vi "IntakeBegin.vi"(8 "error in (no error)":errorcluster) -> (0 "error out":errorcluster)   [LabVIEW 2023]
uses:
  <vilib>/Rock Robotics/WPI/ThirdParty/REV Robotics/REVLib/Typedef/Spark MAX Idle Mode.ctl
  <vilib>/Rock Robotics/SystemInterfaces/DIO/FPGA_DIOChannel.ctl
  <vilib>/Rock Robotics/WPI/ThirdParty/REV Robotics/REVLib/SubVI/Public/SPARK Open Brushless.vi
  <vilib>/Rock Robotics/WPI/ThirdParty/REV Robotics/REVLib/SubVI/Public/SPARK Configure Basic Idle Mode.vi
  <vilib>/Rock Robotics/WPI/Switch/WPI_SwitchOpenLimit.vi
  <vilib>/Rock Robotics/WPI/ThirdParty/REV Robotics/REVLib/SubVI/Public/SPARK Configure Basic Ramp Rate.vi
  <vilib>/Rock Robotics/WPI/ThirdParty/REV Robotics/REVLib/SubVI/Public/SPARK Configure Power Smart Current Limit.vi
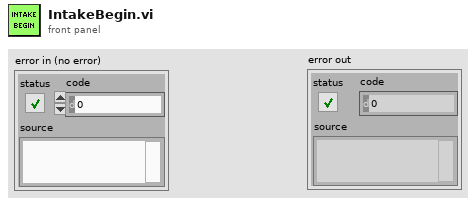
[diagram p1: front panel]
types:
  T1 = typedef "Spark MAX Idle Mode.ctl" = enum16{"Coast", "Brake"}
  T2 = typedef "FPGA_DIOChannel.ctl" = enum8{"DIO 0", "DIO 1", "DIO 2", "DIO 3", "DIO 4", "DIO 5", "DIO 6", "DIO 7", "DIO 8", "DIO 9", "DIO MXP 0", "DIO MXP 1", "DIO MXP 2", "DIO MXP 3", "DIO MXP 4", "DIO MXP 5", "DIO MXP 6", "DIO MXP 7", "DIO MXP 8", "DIO MXP 9", "DIO MXP 10", "DIO MXP 11", "DIO MXP 12", "DIO MXP 13", "DIO MXP 14", "DIO MXP 15", "SPI Port CS1", "SPI Port CS2", "SPI Port CS3", "SPI Port MISO", "SPI Port MOSI", "Invalid"}
  T3 = typedef "WPI_SwitchDevRef.ctl" = cluster{"DevStatus":errorcluster, "DIO Channel":T2, "CntIndex":T4, "Normally Closed":bool}
  T4 = typedef "FPGA_CounterCtrSystemIndex.ctl" = enum8{"Ctr 0", "Ctr 1", "Ctr 2", "Ctr 3", "Ctr 4", "Ctr 5", "Ctr 6", "Ctr 7", "Invalid"}
  T5 = typedef "WPI_MotorControlDeviceRef.ctl" = cluster{"DeviceStatus":errorcluster, "Type":T6, "PWM":cluster{"PWM Channel":T7, "DeadBand":T8}, "CAN":cluster{"Device Number":u8, "SetOutput VI Ref":variant, "GetOutput VI Ref":variant, "Enable VI Ref":variant, "Disable VI Ref":variant, "Data":variant}, "Invert":bool, "DIO PWM":cluster{"PWM \"Enable\" Channel":T7, "DIOChannel":T2, "PWM Rate":dbl}}
  T6 = typedef "WPI_MotorControlType.ctl" = enum16{"PWM", "CAN", "DIO PWM"}
  T7 = typedef "FPGA_DIOPWMChannel.ctl" = enum8{"PWM 0", "PWM 1", "PWM 2", "PWM 3", "PWM 4", "PWM 5", "PWM 6", "PWM 7", "PWM 8", "PWM 9", "PWM MXP 0", "PWM MXP 1", "PWM MXP 2", "PWM MXP 3", "PWM MXP 4", "PWM MXP 5", "PWM MXP 6", "PWM MXP 7", "PWM MXP 8", "PWM MXP 9", "Invalid"}
  T8 = typedef "WPI_PWMDeadband.ctl" = cluster{"Name":string, "maxPositivePwm":i32, "minPositivePwm":i32, "centerPwm":i32, "maxNegativePwm":i32, "minNegativePwm":i32, "angularRange":u16}
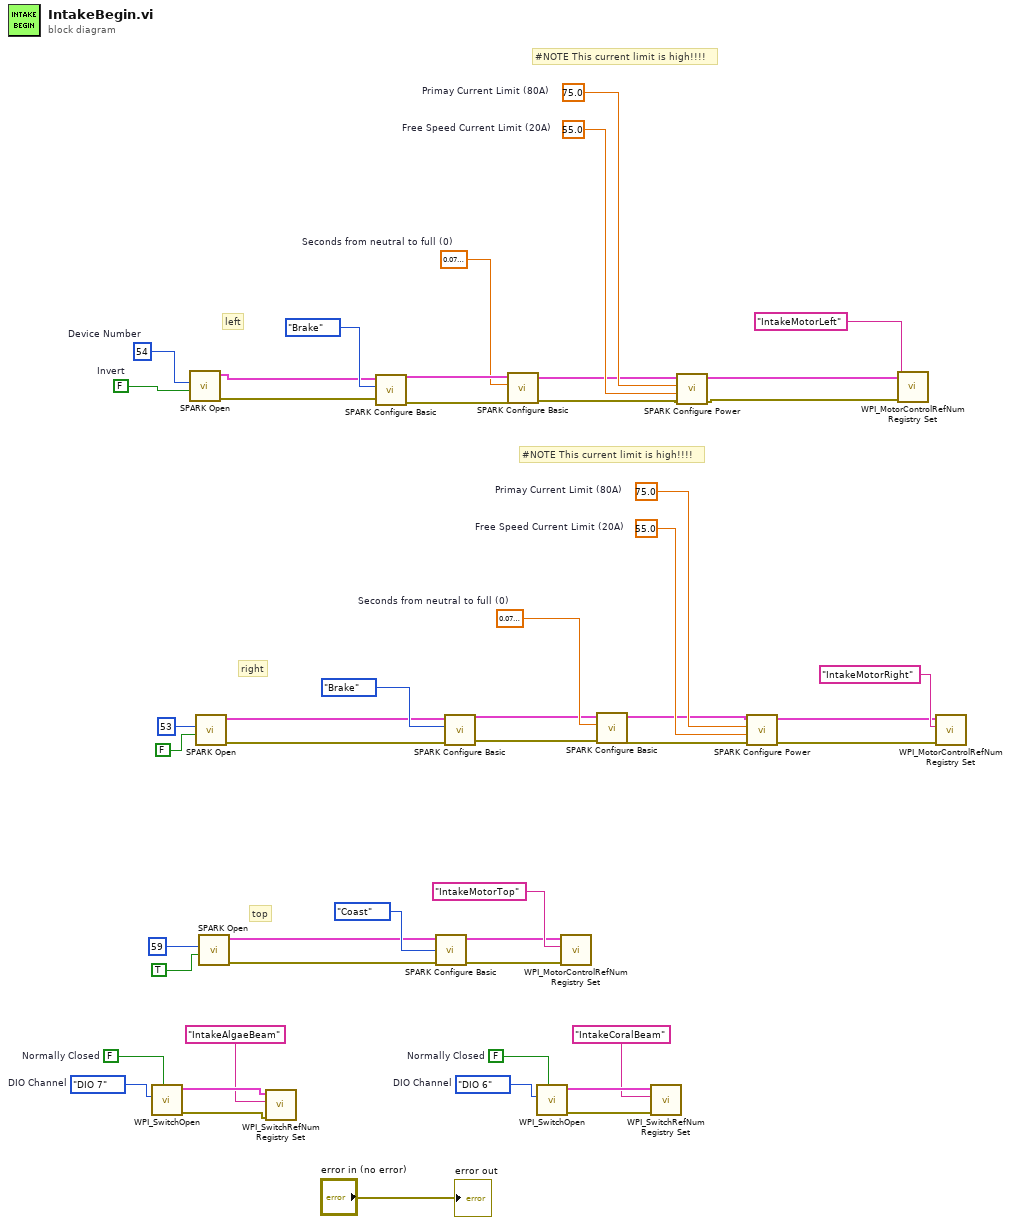
[diagram p0: block diagram]
diagram:
  w13 = sgl 0.08  # Seconds from neutral to full (0)
  w14 = sgl 0.08  # Seconds from neutral to full (0)
  w21 = 55.0  # Free Speed Current Limit (20A)
  w22 = 75.0  # Primay Current Limit (80A)
  w25 = 55.0  # Free Speed Current Limit (20A)
  w26 = 75.0  # Primay Current Limit (80A)
  w30 = FALSE  # Normally Closed
  w31 = FPGA_DIOChannel."DIO 6"  # DIO Channel
  w36 = FALSE  # Normally Closed
  w37 = FPGA_DIOChannel."DIO 7"  # DIO Channel
  w48 = FALSE  # Invert
  w49 = u8 54  # Device Number
  # "top"
  # "#NOTE This current limit is high!!!!"
  # "#NOTE This current limit is high!!!!"
  # "right"
  # "left"
  n1 = call-poly <vilib>:"WPI_SwitchOpen.vi"("Normally Closed"=w36, "DIO Channel"=w37) -> ("error out"=w34:errorcluster, "SwitchDevRef"=w35:T3)  [unwired: 8 in]
  n2 = call-poly <vilib>:"SPARK Open.vi"("Invert"=w48, "Device Number"=w49) -> ("error out"=w40:errorcluster, "MotorControlDeviceRef"=w41:T5)  [unwired: 8 in]
  n3 = call-poly <vilib>:"SPARK Open.vi"("Invert"=FALSE, "Device Number"=u8 53) -> ("error out"=w43:errorcluster, "MotorControlDeviceRef"=w42:T5)  [unwired: 8 in]
  n4 = call-poly <vilib>:"SPARK Open.vi"("Invert"=TRUE, "Device Number"=u8 59) -> ("error out"=w4:errorcluster, "MotorControlDeviceRef"=w5:T5)  [unwired: 8 in]
  n5 = call <vilib>:"WPI_SwitchRefNum Registry Set.vi"("error in (no error)"=w34, "refnum name"="IntakeAlgaeBeam", "SwitchDevRef"=w35) -> ()  [unwired: 7 in, 2 out]
  n6 = call-poly <vilib>:"SPARK Configure Basic.vi"("error in (no error)"=w40, "Idle Mode"=Spark_MAX_Idle_Mode."Brake", "MotorControlDeviceRef in"=w41) -> ("error out"=w17:errorcluster, "MotorControlDeviceRef out"=w18:T5)  [unwired: 7 in]
  n7 = call-poly <vilib>:"SPARK Configure Basic.vi"("error in (no error)"=w4, "Idle Mode"=Spark_MAX_Idle_Mode."Coast", "MotorControlDeviceRef in"=w5) -> ("error out"=w1:errorcluster, "MotorControlDeviceRef out"=w2:T5)  [unwired: 7 in]
  n8 = call-poly <vilib>:"SPARK Configure Basic.vi"("error in (no error)"=w43, "Idle Mode"=Spark_MAX_Idle_Mode."Brake", "MotorControlDeviceRef in"=w42) -> ("error out"=w11:errorcluster, "MotorControlDeviceRef out"=w12:T5)  [unwired: 7 in]
  n9 = call-poly <vilib>:"SPARK Configure Basic.vi"("error in (no error)"=w17, "Seconds from neutral to full (0)"=w14, "MotorControlDeviceRef in"=w18) -> ("error out"=w16:errorcluster, "MotorControlDeviceRef"=w15:T5)  [unwired: 7 in]
  n10 = call-poly <vilib>:"WPI_SwitchOpen.vi"("Normally Closed"=w30, "DIO Channel"=w31) -> ("error out"=w28:errorcluster, "SwitchDevRef"=w29:T3)  [unwired: 8 in]
  n11 = call <vilib>:"WPI_MotorControlRefNum Registry Set.vi"("error in (no error)"=w1, "refnum name"="IntakeMotorTop", "MotorControlDevRef"=w2) -> ()  [unwired: 7 in, 2 out]
  n12 = call-poly <vilib>:"SPARK Configure Basic.vi"("error in (no error)"=w11, "Seconds from neutral to full (0)"=w13, "MotorControlDeviceRef in"=w12) -> ("error out"=w9:errorcluster, "MotorControlDeviceRef"=w10:T5)  [unwired: 7 in]
  n13 = call <vilib>:"WPI_SwitchRefNum Registry Set.vi"("error in (no error)"=w28, "refnum name"="IntakeCoralBeam", "SwitchDevRef"=w29) -> ()  [unwired: 7 in, 2 out]
  n14 = call-poly <vilib>:"SPARK Configure Power.vi"("error in (no error)"=w16, "Free Speed Current Limit (20A)"=w25, "Primay Current Limit (80A)"=w26, "MotorControlDeviceRef in"=w15) -> ("error out"=w23:errorcluster, "MotorControlDeviceRef out"=w24:T5)  [unwired: 6 in]
  n15 = call-poly <vilib>:"SPARK Configure Power.vi"("error in (no error)"=w9, "Free Speed Current Limit (20A)"=w21, "Primay Current Limit (80A)"=w22, "MotorControlDeviceRef in"=w10) -> ("error out"=w19:errorcluster, "MotorControlDeviceRef out"=w20:T5)  [unwired: 6 in]
  n16 = call <vilib>:"WPI_MotorControlRefNum Registry Set.vi"("error in (no error)"=w23, "refnum name"="IntakeMotorLeft", "MotorControlDevRef"=w24) -> ()  [unwired: 7 in, 2 out]
  n17 = call <vilib>:"WPI_MotorControlRefNum Registry Set.vi"("error in (no error)"=w19, "refnum name"="IntakeMotorRight", "MotorControlDevRef"=w20) -> ()  [unwired: 7 in, 2 out]
  "error out" <- "error in (no error)"
